vi "graph error bar simple.vi"(8 "error in":errorcluster, 9 "Yerror 2":dbl[](array[numeric]), 10 "y Values":dbl[](array[numeric]), 11 "x values":dbl[](array[numeric])) -> (0 "error out":errorcluster, 2 "graph out":T1(array[cluster]))   [LabVIEW 2016]
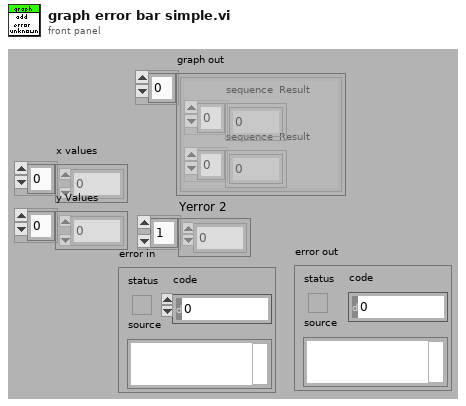
[diagram p1: front panel]
types:
  T1 = cluster{"sequence  Result":dbl[], "sequence  Result":dbl[]}[]
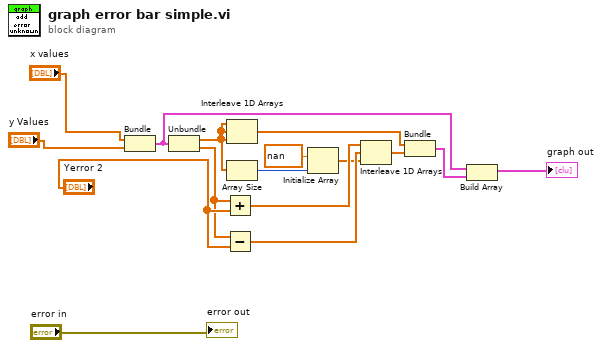
[diagram p0: block diagram]
diagram:
  n1 = Bundle("x values"="x values", "y Values"="y Values") -> (w8:cluster{"x values":dbl[], "y Values":dbl[]})  [unwired: 1 in]
  n2 = Unbundle(w8) -> ("x values"=w5:dbl[], "y Values"=w6:dbl[])
  n3 = Add(x=w6, y="Yerror 2") -> (x+y=w14:dbl[])
  n4 = Subtract(x=w6, y="Yerror 2") -> (x-y=w13:dbl[])
  n5 = Interleave 1D Arrays(w5, w5, w5) -> (w15:dbl[])
  n6 = Array Size(array=w5) -> (size(s)=w12:i32)
  n7 = Initialize Array(nan ("element"), w12) -> (w11:dbl[])
  n8 = Interleave 1D Arrays(w14, w13, w11) -> (w16:dbl[])
  n9 = Bundle(w15, w16) -> (w9:cluster{dbl[], dbl[]})  [unwired: 1 in]
  n10 = Build Array(w8, w9) -> (→"graph out":cluster{"x values":dbl[], "y Values":dbl[]}[])
  "error out" <- "error in"
